vi "2100_HV Load Test w_Telegram Write and Source Delay.vi"(0 "Semiconductor Module Context":T3, 1 "Reg0_State":string="State00", 2 "HSDIO_Pins":string[](array[string])=["CLK", "SDA"], 3 "Published_Data_ID":string="HV39_", 5 "HV_Load_Steps_uA":dbl[](array[numeric])=[0.0, 5.0, 8.0, 10.0] format="%#_6p", 7 "USID":T2 max=15, 9 "Reg_Address_Data":T1={"Address"=10, "Data"=133} {"Address" format="%.0x"}, 11 "error in (no error)":errorcluster, 12 "Num_Of_Telegrams":i32=100) -> (15 "error out":errorcluster)   [LabVIEW 2013]
uses:
  <vilib>/NI_TestStand_SemiconductorModule/NI_TestStand_Semiconductor_Module.lvlibp/PinMap/General/SemiconductorModuleContext.ctl
  Controls/USID.ctl
  Controls/Reg_Address_Data.ctl
  <instrlib>/niDCPower/nidcpower.llb/niDCPower Measurement Type.ctl
  <vilib>/NI_TestStand_SemiconductorModule/NI_TestStand_Semiconductor_Module.lvlibp/PinMap/DC Power/PinsToNIDCPowerSessions.vi
  <vilib>/NI_TestStand_SemiconductorModule/NI_TestStand_Semiconductor_Module.lvlibp/PinMap/Deprecated/PublishDataDoubleMultiplePinsSingleInstrument.vi
  <vilib>/NI_TestStand_SemiconductorModule/NI_TestStand_Semiconductor_Module.lvlibp
panel:
  in  "Measurement:Aperture Time":dbl
  in  "Source:Advanced:Source Delay":dbl=2.5e-05 format="%#_13p"
  in  "Source:Transient Response":i32(ring)=1041 items=["Slow"=1041, "Normal"=1038, "Fast"=1039, "Custom"=1042]
  out "Immediate Current Measurements":dbl[][](array[numeric]) format="%#_6p"
  out "Default Source Delay":dbl[](array[numeric])
  out "current measurements":dbl[][](array[numeric]) format="%#_6p"
  out "voltage measurements":dbl[][](array[numeric])
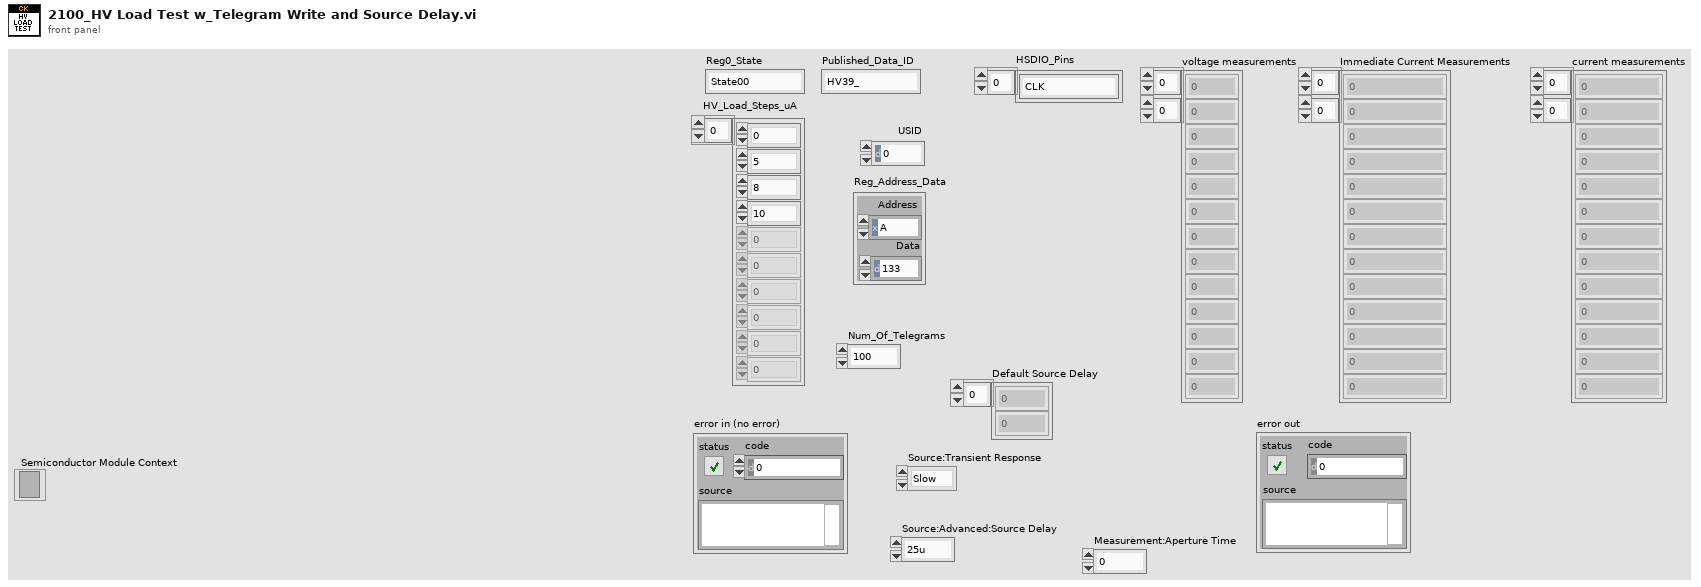
[diagram p1: front panel]
types:
  T1 = typedef "Reg_Address_Data.ctl" = cluster{"Address":u8, "Data":u8}
  T2 = typedef "USID.ctl" = u8
  T3 = typedef "NI_TestStand_Semiconductor_Module.lvlibp/SemiconductorModuleContext.ctl" = refnum<k7>
  T4 = typedef "niDCPower Measurement Type.ctl" = i32
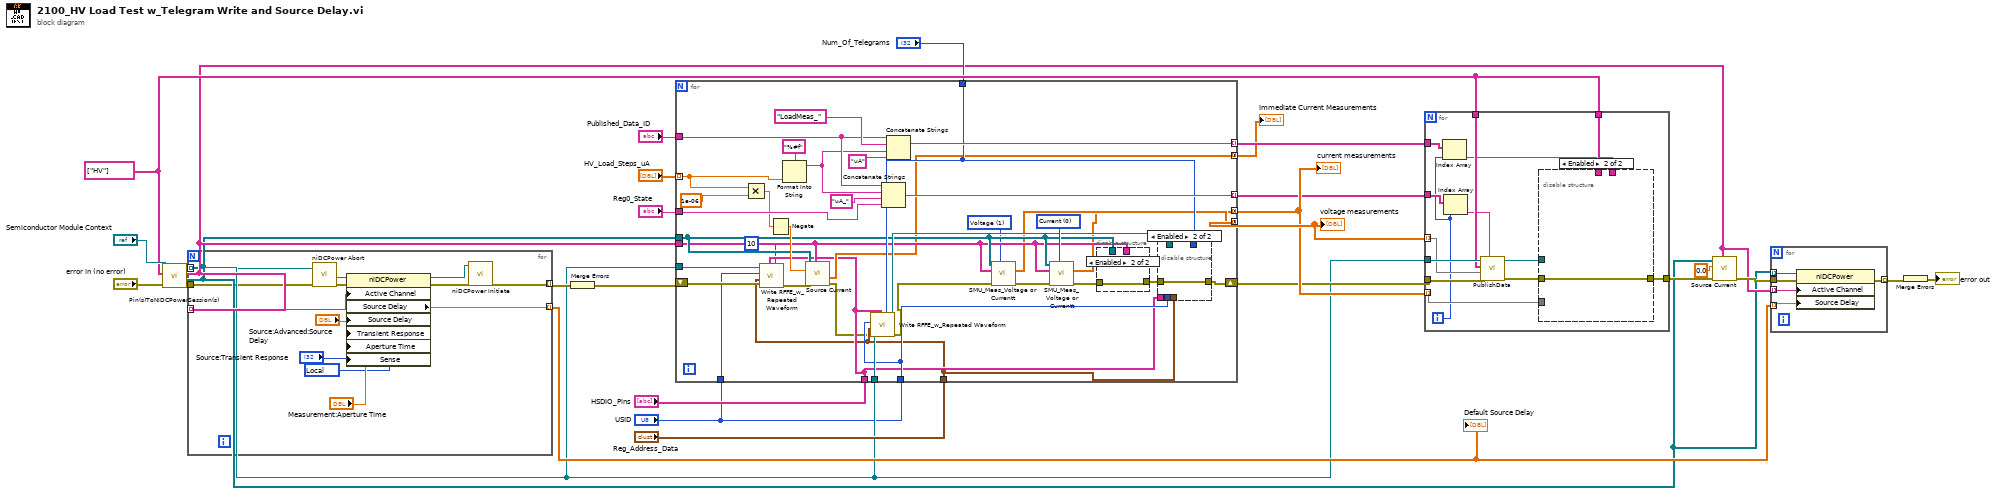
[diagram p0: block diagram]
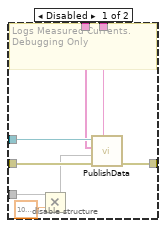
[diagram p2: hidden frame]
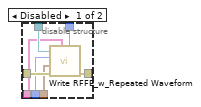
[diagram p3: hidden frame]
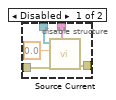
[diagram p4: hidden frame]
diagram:
  w22 = string[] ["HV"] ("Pins")
  n1 = call-poly <vilib>:"Pin(s)ToNIDCPowerSession(s).vi"("error in (no error)"="error in (no error)", "Pins"=w22, "Semiconductor Module Context"="Semiconductor Module Context") -> ("error out"=w11:errorcluster, "Instrument Sessions"=w5:refnum<k15>[], "Channel Lists"=w6:string[], "Semiconductor Module Context Out"=w2:T3)  [unwired: 4 in, 1 out]
  n2 = for {
    tunnel: w6 -> [w41] mode=indexing
    tunnel: w5 -> [w35] mode=indexing
    tunnel: w11 -> [w38]
    tunnel: [w33] -> w10 mode=indexing
    tunnel: [w39] -> w8 mode=indexing
    w29 = 1008 items=["Local"=1008, "Remote"=1009] ("Measurement:Sense")
    n3 = call <instrlib>:"niDCPower Abort.vi"("error in (no error)"=w38, "instrument handle"=w35) -> ("error out"=w37:errorcluster, "instrument handle out"=w36:refnum<k15>)  [unwired: 8 in]
    n4 = property class="niDCPower"(reference=w36, error in=w37, "Active Channel"=w41, "Source Delay"="Source:Advanced:Source Delay", "Transient Response"="Source:Transient Response", "Aperture Time"="Measurement:Aperture Time", "Sense"=w29) -> (reference out=w32:refnum<k15>, error out=w34:errorcluster, "Source Delay"=w39:dbl)
    n5 = call <instrlib>:"niDCPower Initiate.vi"("error in (no error)"=w34, "instrument handle"=w32) -> ("error out"=w33:errorcluster)  [unwired: 8 in, 1 out]
  }
  "Default Source Delay" <- w8
  n6 = Merge Errors(w10) -> (w9:errorcluster)
  n7 = for {
    tunnel: w6 -> [w55]
    tunnel: "HV_Load_Steps_uA" -> [w67] mode=indexing
    tunnel: w5 -> [w56]
    shift-right: [w61] -> w15
    shift-left: w9 -> [w50]
    tunnel: "Published_Data_ID" -> [w73]
    tunnel: "Reg0_State" -> [w76]
    tunnel: [w52] -> w23 mode=concatenating
    tunnel: [w75] -> w18 mode=indexing
    tunnel: [w51] -> w21 mode=concatenating
    tunnel: [w72] -> w19 mode=indexing
    tunnel: w2 -> [w65]
    tunnel: "HSDIO_Pins" -> [w48]
    tunnel: "USID" -> [w59]
    tunnel: "Reg_Address_Data" -> [w45]
    tunnel: "Num_Of_Telegrams" -> [w58]
    tunnel: [w53] -> w3 mode=concatenating
    tunnel: w2 -> [w47]
    tunnel: "USID" -> [w46]
    w54 = T4 1 items=["Current", "Voltage"] ("measurement type")
    w64 = T4 0 items=["Current", "Voltage"] ("measurement type")
    n8 = Multiply(x=w67, y=1e-06) -> (x*y=w69:dbl)
    n9 = call "Write RFFE_w_Repeated Waveform.vi"("Num_Of_Telegrams"=10, "Pins"=w48, "error in (no error)"=w50, "Reg_Address_Data"=w45, "USID"=w46, "Semiconductor Module Context"=w47) -> ("error out"=w49:errorcluster)  [unwired: 4 in, 1 out]
    n10 = Negate(x=w69) -> (-x=w77:dbl)
    n11 = Format Into String(format string="%#f", w67) -> (resulting string=w66:string)  [unwired: 2 in, 1 out]
    n12 = call "Source Current.vi"("Channel Lists"=w55, "error in (no error)"=w49, "current level"=w77, "Instrument Sessions In"=w56) -> ("error out"=w43:errorcluster, "current measurements"=w53:dbl[][])  [unwired: 4 in, 2 out]
    n13 = call "Write RFFE_w_Repeated Waveform.vi"("Num_Of_Telegrams"=w58, "Pins"=w48, "error in (no error)"=w43, "Reg_Address_Data"=w45, "USID"=w59, "Semiconductor Module Context"=w65) -> ("error out"=w42:errorcluster, "Semiconductor Module Context Out"=w60:T3)  [unwired: 4 in]
    n14 = Concatenate Strings(w73, w66, "uA_" ("string"), w76) -> (w75:string)
    n15 = Concatenate Strings(w73, "LoadMeas_" ("string"), w66, "uA" ("string")) -> (w72:string)
    n16 = call "SMU_Meas_Voltage or Currentt.vi"("measurement type"=w54, "error in (no error)"=w42, "Channel Lists"=w55, "DCPower Sessions In"=w56) -> ("error out"=w57:errorcluster, "Measurement"=w52:dbl[][])  [unwired: 5 in, 1 out]
    n17 = call "SMU_Meas_Voltage or Currentt.vi"("measurement type"=w64, "error in (no error)"=w57, "Channel Lists"=w55, "DCPower Sessions In"=w56) -> ("error out"=w63:errorcluster, "Measurement"=w51:dbl[][])  [unwired: 5 in, 1 out]
    n18 = disable-structure shown="Enabled" {
      disable-tunnel: w63 -> [w91 w92]
      disable-tunnel: [w89 w92] -> w62
      disable-tunnel: w56 -> [w88 _]
      disable-tunnel: w55 -> [w87 _]
      frame Disabled {
        n19 = call "Source Current.vi"("Channel Lists"=w87, "error in (no error)"=w91, "current level"=0.0, "Instrument Sessions In"=w88) -> ("error out"=w89:errorcluster)  [unwired: 4 in, 3 out]
      }
      frame Enabled {
      }
    }
    n20 = disable-structure shown="Enabled" {
      disable-tunnel: w62 -> [w85 w86]
      disable-tunnel: [w84 w86] -> w61
      disable-tunnel: w45 -> [w83 _]
      disable-tunnel: w60 -> [w82 _]
      disable-tunnel: w59 -> [w81 _]
      disable-tunnel: w48 -> [w80 _]
      disable-tunnel: w58 -> [w79 _]
      frame Disabled {
        n21 = call "Write RFFE_w_Repeated Waveform.vi"("Num_Of_Telegrams"=w79, "Pins"=w80, "error in (no error)"=w85, "Reg_Address_Data"=w83, "USID"=w81, "Semiconductor Module Context"=w82) -> ("error out"=w84:errorcluster)  [unwired: 4 in, 1 out]
      }
      frame Enabled {
      }
    }
  }
  "voltage measurements" <- w23
  "current measurements" <- w21
  "Immediate Current Measurements" <- w3
  n22 = for {
    tunnel: w15 -> [w106]
    tunnel: [w102] -> w24
    tunnel: w2 -> [w105]
    tunnel: w23 -> [w104] mode=indexing
    tunnel: w22 -> [w103]
    tunnel: w22 -> [w99]
    tunnel: w21 -> [w98] mode=indexing
    tunnel: w18 -> [w97]
    tunnel: w19 -> [w96]
    i -> [w93]
    n23 = Index Array(array=w96, index=w93) -> (element=w95:string)
    n24 = Index Array(array=w97, index=w93) -> (element=w94:string)
    n25 = call-poly <vilib>:"PublishData.vi"("Measurement Id"=w94, "error in (no error)"=w106, "Data In"=w104, "Pins"=w103, "Semiconductor Module Context"=w105) -> ("error out"=w101:errorcluster, "Semiconductor Module Context Out"=w100:T3)  [unwired: 5 in]
    n26 = disable-structure shown="Enabled" {
      disable-tunnel: [w114 w115] -> w102
      disable-tunnel: w101 -> [w113 w115]
      disable-tunnel: w100 -> [w112 _]
      disable-tunnel: w99 -> [w111 _]
      disable-tunnel: w98 -> [w108 _]
      disable-tunnel: w95 -> [w107 _]
      frame Disabled {
        # "Logs Measured Currents.\nDebugging Only"
        n27 = Multiply(x=w108, y=1000000.0) -> (x*y=w110:dbl[])
        n28 = call-poly <vilib>:"PublishData.vi"("Measurement Id"=w107, "error in (no error)"=w113, "Data In"=w110, "Pins"=w111, "Semiconductor Module Context"=w112) -> ("error out"=w114:errorcluster)  [unwired: 5 in, 1 out]
      }
      frame Enabled {
      }
    }
  }
  n29 = call "Source Current.vi"("Channel Lists"=w6, "error in (no error)"=w24, "current level"=0.0, "Instrument Sessions In"=w5) -> ("error out"=w7:errorcluster)  [unwired: 4 in, 3 out]
  n30 = for {
    tunnel: w8 -> [w119] mode=indexing
    tunnel: [w120] -> w4 mode=indexing
    tunnel: w7 -> [w118]
    tunnel: w6 -> [w117] mode=indexing
    tunnel: w5 -> [w116] mode=indexing
    n31 = property class="niDCPower"(reference=w116, error in=w118, "Active Channel"=w117, "Source Delay"=w119) -> (error out=w120:errorcluster)  [unwired: 1 out]
  }
  n32 = Merge Errors(w4) -> (→"error out":errorcluster)
